vi "SSH OpenSSH Session FGV.vi"(8 "error in (no error)":errorcluster, 10 "OpenSSH Session Op":T1, 11 "OpenSSH Client in":refnum<class "OpenSSH Client.lvclass">) -> (0 "error out":errorcluster, 3 "OpenSSH Client out":refnum<class "OpenSSH Client.lvclass">)   [LabVIEW 2024, in "LMH-LINX.lvlib"]
uses:
  <vilib>/MakerHub/LINX/LMH-LINX.lvlib
  <vilib>/net/SSH/Client/OpenSSH/OpenSSH Client.lvclass
  <vilib>/MakerHub/LINX/Private/Utilties/SSH/SSH OpenSSH Session Op.ctl
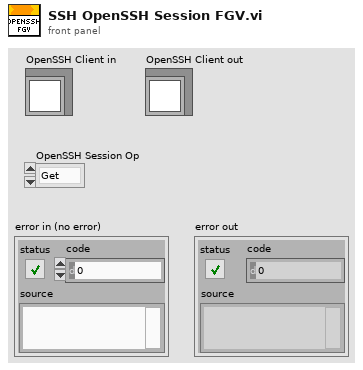
[diagram p1: front panel]
types:
  T1 = typedef "LMH-LINX.lvlib/SSH OpenSSH Session Op.ctl" = enum16{"Get", "Set"}
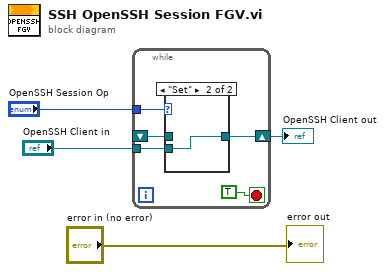
[diagram p0: block diagram]
diagram:
  n1 = while {
    shift-right: [w6] -> w2
    shift-left: _ -> [w5]
    tunnel: "OpenSSH Session Op" -> [w8]
    tunnel: "OpenSSH Client in" -> [w7]
    stop <- TRUE stop-if-true
    n2 = case shown="\"Set\"" w8 {
      tunnel: w7 -> [_ w11]
      tunnel: [w10 w11] -> w6
      tunnel: w5 -> [w10 _]
      frame "Get", Default {
      }
      frame "Set" {
      }
    }
  }
  "OpenSSH Client out" <- w2
  "error out" <- "error in (no error)"
